vi "Convert Key Value Pairs to Log Row.vi"(8 "error in (no error)":errorcluster, 10 "Key Value Pairs":T1[](array[typedef]), 11 "Headers In[]":string[](array[string])) -> (0 "error out":errorcluster, 2 "Data Out[]":string[](array[string]), 3 "Headers Out[]":string[](array[string]))   [LabVIEW 2016, in "SLL Spreadsheet.lvlib" / "SLL CSV Logger.lvclass"]
uses:
  SLL CSV Logger.lvclass
  _Typedefs/String Key Value Pair Cluster.ctl
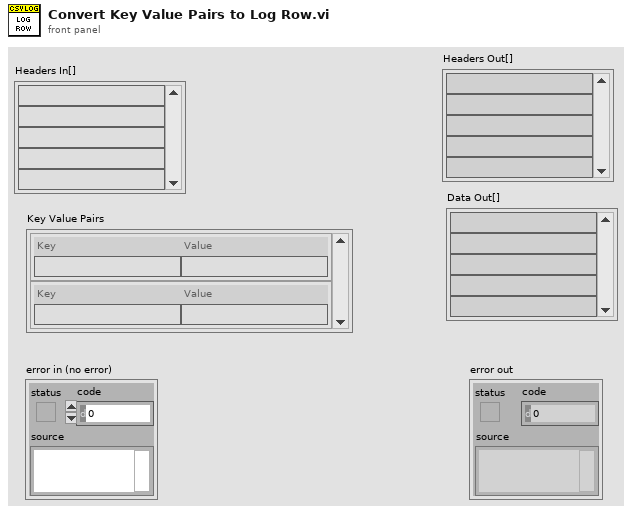
[diagram p1: front panel]
types:
  T1 = typedef "SLL Spreadsheet.lvlib/SLL CSV Logger.lvclass/String Key Value Pair Cluster.ctl" = cluster{"Key":string, "Value":string}
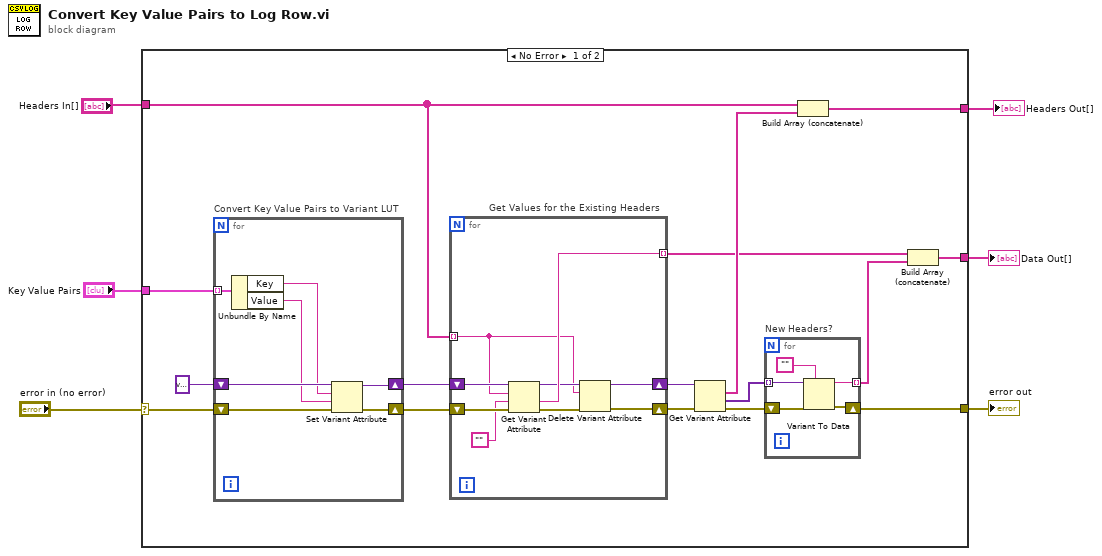
[diagram p0: block diagram]
diagram:
  n1 = case shown="No Error" "error in (no error)" {
    selector: "error in (no error)" -> [w20 w45]
    tunnel: [w10 w45] -> w5
    tunnel: "Headers In[]" -> [w15 w44]
    tunnel: "Key Value Pairs" -> [w22 _]
    tunnel: [w13 w44] -> w2
    tunnel: [w7 _] -> w1
    frame No Error {
      n2 = for "Convert Key Value Pairs to Variant LUT" {
        tunnel: w22 -> [w41] mode=indexing
        shift-right: [w42] -> w18
        shift-left: variant ("variant") -> [w43]
        shift-right: [w37] -> w19
        shift-left: w20 -> [w38]
        n3 = Unbundle By Name(w41) -> ("Key"=w40:string, "Value"=w39:string)
        n4 = Set Variant Attribute(Variant=w43, name=w40, value=w39, error in=w38) -> (Variant out=w42:variant, error out=w37:errorcluster)  [unwired: 1 out]
      }
      n5 = for "Get Values for the Existing Headers" {
        tunnel: w15 -> [w28] mode=indexing
        shift-right: [w29] -> w17
        shift-left: w18 -> [w35]
        tunnel: [w33] -> w9 mode=indexing
        shift-right: [w30] -> w16
        shift-left: w19 -> [w36]
        n6 = Get Variant Attribute(Variant=w35, name=w28, default value (empty Variant)="", error in=w36) -> (duplicate Variant=w32:variant, value=w33:string, error out=w31:errorcluster)  [unwired: 1 out]
        n7 = Delete Variant Attribute(4:w31, 6:w28, 7:w32) -> (0:w30:errorcluster, 3:w29:variant)  [unwired: 1 out]
      }
      n8 = Get Variant Attribute(Variant=w17, error in=w16) -> (names=w14:string[], values=w12:variant[], error out=w11:errorcluster)  [unwired: 2 in, 1 out]
      n9 = for "New Headers?" {
        tunnel: w12 -> [w27] mode=indexing
        shift-right: [w25] -> w10
        shift-left: w11 -> [w26]
        tunnel: [w23] -> w8 mode=indexing
        n10 = Variant To Data(error in=w26, type="", Variant=w27) -> (data=w23:string, error out=w25:errorcluster)
      }
      n11 = Build Array (concatenate)(w15, w14) -> (w13:string[])
      n12 = Build Array (concatenate)(w9, w8) -> (w7:string[])
    }
    frame Error {
    }
  }
  "error out" <- w5
  "Headers Out[]" <- w2
  "Data Out[]" <- w1
